vi "Refresh CO Terminal.vi"(10 "错误输入（无错误）":errorcluster, 11 "Status":T1 {"Setting"."X Pos." scale=-2.0..2.0; "Setting"."Y Pos." scale=-2.0..2.0}) -> (2 "错误输出":errorcluster)   [LabVIEW 2013]
uses:
  init-status.ctl
  Setting.ctl
  event-package.ctl
  Event1.ctl
  data-package.ctl
  Event.ctl
  <vilib>/DAQmx/create/channels.llb/DAQmx Create Channel (CO-Pulse Generation-Frequency).vi
  <vilib>/DAQmx/configure/timing.llb/DAQmx Timing (Implicit).vi
  <vilib>/DAQmx/create/channels.llb/DAQmx Create Channel (AO-Voltage-Basic).vi
  <vilib>/DAQmx/create/channels.llb/DAQmx Create Channel (AI-Voltage-Basic).vi
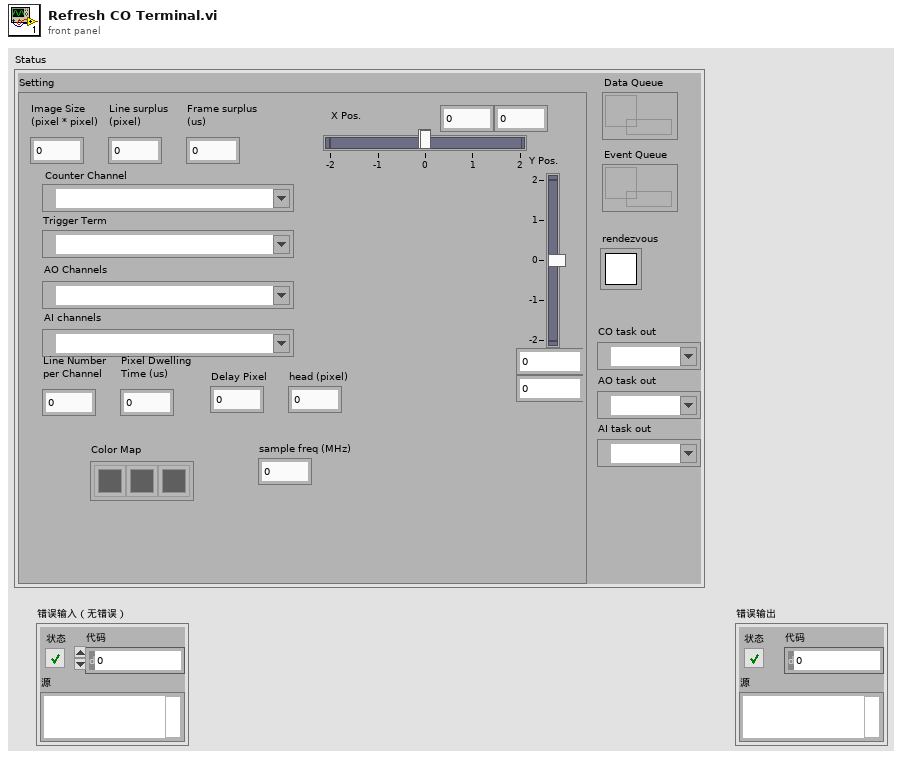
[diagram p1: front panel]
types:
  T1 = typedef "init-status.ctl" = cluster{"Setting":T2, "Event Queue":refnum<queue>, "Data Queue":refnum<queue>, "rendezvous":T3, "CO task out":refnum<k21>, "AO task out":refnum<k21>, "AI task out":refnum<k21>}
  T2 = typedef "Setting.ctl" = cluster{"Image Size\n(pixel * pixel)":i32, "Counter Channel":tag, "Trigger Term":tag, "AO Channels":tag, "Y Pos.":cluster{dbl, dbl}, "X Pos.":cluster{dbl, dbl}, "Line surplus\n(pixel)":i32, "Frame surplus\n(us)":i32, "AI channels":tag, "Line Number\nper Channel":i32, "Delay Pixel":i32, "Pixel Dwelling\nTime (us)":i32, "Color Map":u32[], "head (pixel)":i32, "sample freq (MHz)":dbl}
  T3 = typedef "Rendezvous RefNum" = refnum<k1>
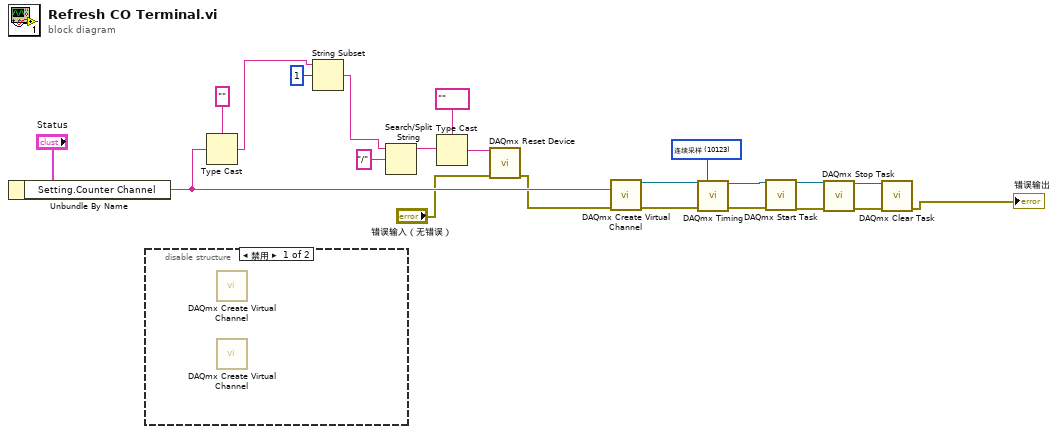
[diagram p0: block diagram]
diagram:
  w19 = 10123 items=["有限采样"=10178, "连续采样"=10123, "硬件定时单点"=12522] ("sample mode")
  n1 = Unbundle By Name("Status") -> ("Setting.Counter Channel"=w18:tag)
  n2 = disable-structure shown="禁用" {
    frame Disabled {
      n3 = call-poly <vilib>:"DAQmx Create Virtual Channel.vi"() -> ()  [unwired: 14 in, 2 out]
      n4 = call-poly <vilib>:"DAQmx Create Virtual Channel.vi"() -> ()  [unwired: 14 in, 2 out]
    }
    frame Enabled {
    }
  }
  n5 = Type Cast(type="", x=w18) -> (*(type *) &x=w1:string)
  n6 = String Subset(string=w1, offset (0)=1 ("偏移量(0)")) -> (substring=w2:string)  [unwired: 1 in]
  n7 = Search/Split String(string=w2, search string/char (-)="/" ("搜索字符串/字符(-)")) -> (substring before match=w4:string)  [unwired: 1 in, 2 out]
  n8 = Type Cast(type=tag "" ("device in"), x=w4) -> (*(type *) &x=w7:tag)
  n9 = call <vilib>:"DAQmx Reset Device.vi"("device in"=w7, "error in"="错误输入（无错误）") -> ("error out"=w5:errorcluster)  [unwired: 13 in]
  n10 = call-poly <vilib>:"DAQmx Create Virtual Channel.vi"("counter"=w18, "error in"=w5) -> ("task out"=w20:refnum<k21>, "error out"=w21:errorcluster)  [unwired: 12 in]
  n11 = call-poly <vilib>:"DAQmx Timing.vi"("task/channels in"=w20, "sample mode"=w19, "error in"=w21) -> ("task out"=w15:refnum<k21>, "error out"=w12:errorcluster)  [unwired: 11 in]
  n12 = call <vilib>:"DAQmx Start Task.vi"("task/channels in"=w15, "error in"=w12) -> ("task out"=w14:refnum<k21>, "error out"=w13:errorcluster)  [unwired: 12 in]
  n13 = call <vilib>:"DAQmx Stop Task.vi"("task/channels in"=w14, "error in"=w13) -> ("task out"=w17:refnum<k21>, "error out"=w16:errorcluster)  [unwired: 12 in]
  n14 = call <vilib>:"DAQmx Clear Task.vi"("task in"=w17, "error in"=w16) -> ("error out"=→"错误输出":errorcluster)  [unwired: 13 in]
